vi "Configure Read Memory.vi"(8 "error in (no error)":errorcluster, 9 "Last Read No.":i32 min=0 max=99999 format="%#.6g", 10 "First Read No.":i32 min=0 max=9999 format="%#.6g", 11 "VISA resource name":refnum<visa-resource-name>) -> (0 "error out":errorcluster, 2 "Count":u32, 3 "VISA resource name out":refnum<visa-resource-name>)   [LabVIEW 2017, in "ADCMT7451_ADC.lvlib"]
doc: "Configures to read measurement data memory."
uses:
  ADCMT7451_ADC.lvlib
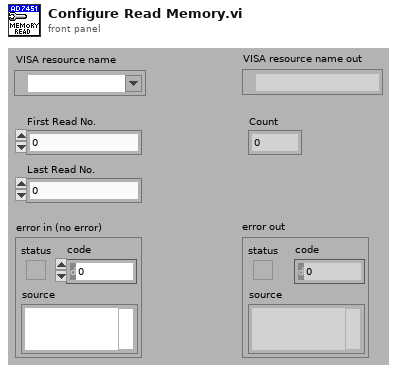
[diagram p1: front panel]
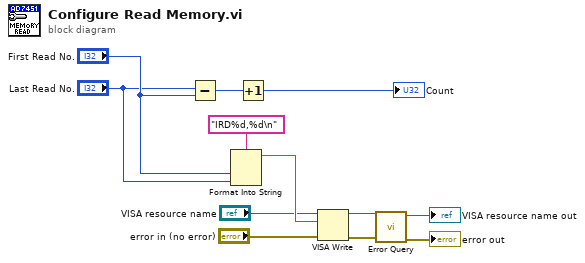
[diagram p0: block diagram]
diagram:
  n1 = Subtract(x="Last Read No.", y="First Read No.") -> (x-y=w4:i32)
  n2 = Format Into String(format string="IRD%d,%d\n", "First Read No.", "Last Read No.") -> (resulting string=w9:string)  [unwired: 2 in, 1 out]
  n3 = Increment(x=w4) -> (x+1=→"Count":i32)
  n4 = VISA Write(VISA resource name="VISA resource name", write buffer=w9, error in (no error)="error in (no error)") -> (VISA resource name out=w3:refnum<visa-resource-name>, error out=w2:errorcluster)  [unwired: 1 out]
  n5 = call "Error Query.vi"("error in (no error)"=w2, "VISA resource name"=w3) -> ("error out"=→"error out":errorcluster, "VISA resource name out"=→"VISA resource name out":refnum<visa-resource-name>)  [unwired: 6 in, 2 out]
